vi "Test Gets Rid of Old Received.vi"() -> ()   [LabVIEW 2020, in "Basic.Mechanics.Tests.lvclass"]
uses:
  Basic.Mechanics.Tests.lvclass
  Source/Approval Tests/Options/Options.lvclass
  Source/Approval Tests/Report Nothing/Report Nothing.lvclass
  C:/Users/SAS/Desktop/ApprovalTests.LabVIEW/Source/Approval Tests/Reporter/Reporter.lvclass
  Source/Approval Tests/Options/Options.lvclass/Options.ctl
  Source/Approval Tests/Naming Data/Naming Data.lvclass/Naming Data.ctl
  d27a92d8-1944-4452-9057-093efe2cb2fc.vi
  Source/Approval Tests/Options/Write Reporter.vi
  d27a92d8-1944-4452-9057-093efe2cb2fc.vi/93c5622b-9fb7-41e0-8c76-3fde37e94e34.vi
  Source/Approval Tests/Verify Core.vi
  Source/Approval Tests/Update Test Name if Not Defined.vi
  Source/Approval Tests/Options/Read Scrubber.vi
  d27a92d8-1944-4452-9057-093efe2cb2fc.vi/93c5622b-9fb7-41e0-8c76-3fde37e94e34.vi/04cb982b-2eda-40d0-8d7e-90f8e0b569b2.vi
  Source/Approval Tests/Options/Read Namer.vi
  Source/Approval Tests/Options/Read Naming Data.vi
  Source/Approval Tests/Options/Read Reporter.vi
  Source/Approval Tests/Naming Data/Read Test VI Name.vi
  Source/Approval Tests/Naming Data/Write Test VI Name.vi
  Source/Approval Tests/conv EOL.vi
  Source/Approval Tests/Reporter/Report.vi
  <vilib>/addons/_JKI Toolkits/Caraya/classes/Assert/Assert True.vi
  <vilib>/addons/_JKI Toolkits/Caraya/classes/Assert/Assert False.vi
  <vilib>/addons/_JKI Toolkits/Caraya/classes/Assert/Assert Equal Value_Variant.vi
  Source/Approval Tests/Scrubber/Scrubber.lvclass
  Source/Approval Tests/Namer/Namer.lvclass
  Source/Approval Tests/Naming Data/Naming Data.lvclass
  Source/Approval Tests/Reporter/Reporter.lvclass
  Basic.Mechanics.Tests.lvclass/Basic.Mechanics.Tests.ctl
  <vilib>/addons/_JKI Toolkits/Caraya/classes/Test/Test.lvclass
  <vilib>/addons/_JKI Toolkits/Caraya/classes/Assert/Assert.lvclass
panel:
  out "error out":errorcluster
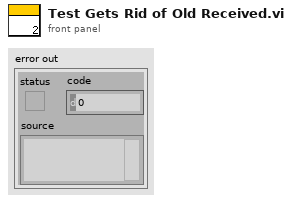
[diagram p1: front panel]
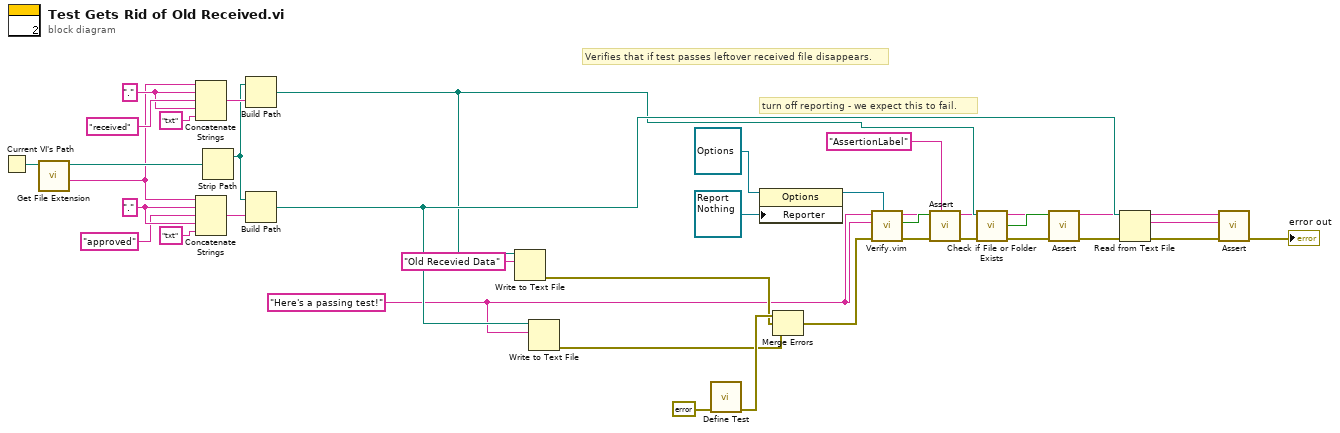
[diagram p0: block diagram]
diagram:
  w21 = "." ("string")
  w26 = "." ("string")
  w1 = "Here's a passing test!"
  # "turn off reporting - we expect this to fail."
  # "Verifies that if test passes leftover received file disappears."
  n1 = Current VI's Path() -> (path=w28:path)
  n2 = call <vilib>:"Get File Extension.vi"("file"=w28) -> ("filename without extension"=w20:string, "dup file"=w27:path)  [unwired: 6 in, 3 out]
  n3 = Concatenate Strings(w20, w21, "received" ("string"), w21, "txt" ("string")) -> (w23:string)
  n4 = Concatenate Strings(w20, w26, "approved" ("string"), w26, "txt" ("string")) -> (w24:string)
  n5 = Strip Path(path=w27) -> (stripped path=w15:path)  [unwired: 1 out]
  n6 = Build Path(base path=w15, name or relative path=w23) -> (appended path=w3:path)
  n7 = Build Path(base path=w15, name or relative path=w24) -> (appended path=w8:path)
  n8 = Write to Text File(file (use dialog)=w3, text="Old Recevied Data") -> (error out=w6:errorcluster)  [unwired: 2 in, 2 out]
  n9 = Write to Text File(file (use dialog)=w8, text=w1) -> (error out=w7:errorcluster)  [unwired: 2 in, 2 out]
  n10 = call <vilib>:"Define Test.vi"("error in (no error)"=errorcluster {"status"=FALSE, "code"=0, "source"=""}) -> ("error out"=w9:errorcluster)  [unwired: 9 in, 1 out]
  n11 = property on="Property Node" class="Options"(reference=refnum<class "Options.lvclass"> refnum ("Options"), "Reporter"=refnum<class "Report Nothing.lvclass"> refnum ("Approval Tests.lvlib:Report Nothing")) -> (reference out=w33:refnum<class "Options.lvclass">)  [unwired: 1 in, 1 out]
  n12 = Merge Errors(w9, w6, w7) -> (w12:errorcluster)
  n13 = call "Verify.vim"("Options"=w33, "error in"=w12, "Anything"=w1) -> ("error out"=w11:errorcluster, "Passed?"=w29:bool)  [unwired: 6 in, 1 out]
  n14 = call-poly <vilib>:"Assert.vi"("Label"="AssertionLabel" ("Label (VI Title)"), "error in (no error)"=w11, "True?"=w29) -> ("error out"=w5:errorcluster)  [unwired: 7 in, 1 out]
  n15 = call <vilib>:"Check if File or Folder Exists.vi"("error in (no error)"=w5, "path"=w3) -> ("error out"=w4:errorcluster, "file or folder exists?"=w2:bool)  [unwired: 7 in, 1 out]
  n16 = call-poly <vilib>:"Assert.vi"("error in (no error)"=w4, "False?"=w2) -> ("error out"=w19:errorcluster)  [unwired: 8 in, 1 out]
  n17 = Read from Text File(file (use dialog)=w8, error in=w19) -> (text=w17:string, error out=w18:errorcluster)  [unwired: 2 in, 2 out]
  n18 = call-poly <vilib>:"Assert.vi"("error in (no error)"=w18, "Y"=w17, "X"=w1) -> ("error out"=→"error out":errorcluster)  [unwired: 7 in, 1 out]
